vi "Verify Checksum.vi"(6 "error in (no error)":errorcluster, 8 "Input Cmd":string) -> (0 "error out":errorcluster, 2 "Trimmed String":string)   [LabVIEW 2013, in "TDK-Lambda Z.lvlib"]
doc: "This VI will add a checksum to any command string.\nThe format of the \"ChkSum Cmd\" output is:\n \"Command\" & \"Dollar Sign\" & \"Two Hex Digits\" & \"Carriage Return\"\n\nThe command is only formulated, it is not sent to the instrument.\n\nVerify the \"$xx\" checksum which was appended to end of any response string"
uses:
  TDK-Lambda Z.lvlib
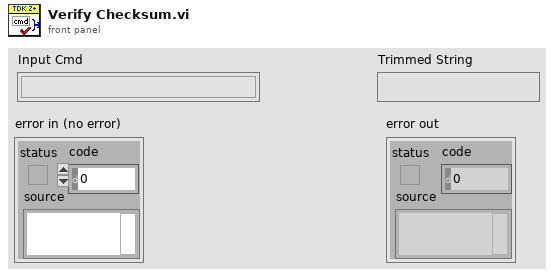
[diagram p1: front panel]
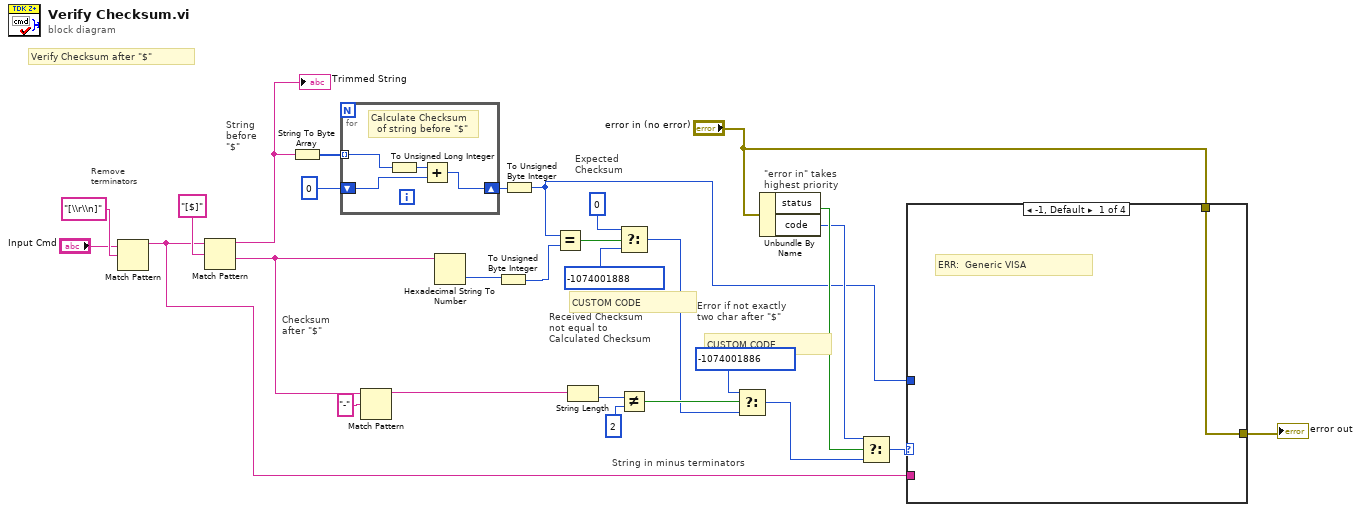
[diagram p0: block diagram]
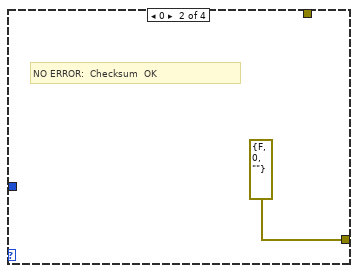
[diagram p2: hidden frame]
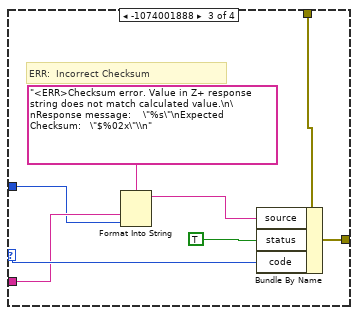
[diagram p3: hidden frame]
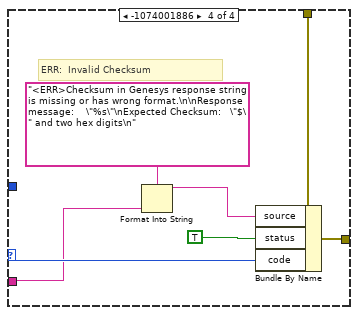
[diagram p4: hidden frame]
diagram:
  # "Expected\nChecksum"
  # "String in minus terminators"
  # "\"error in\" takes\nhighest priority"
  # "String\nbefore\n\"$\""
  # "Checksum\nafter \"$\""
  # "CUSTOM CODE"
  # "Received Checksum\nnot equal to\nCalculated Checksum"
  # "Error if not exactly\ntwo char after \"$\""
  # "CUSTOM CODE"
  # "Remove\nterminators"
  # "Verify Checksum after \"$\""
  n1 = Match Pattern(string="Input Cmd", regular expression="[\\r\\n]") -> (before substring=w9:string)  [unwired: 1 in, 3 out]
  n2 = Match Pattern(string=w9, regular expression="[$]") -> (before substring=w10:string, after substring=w3:string)  [unwired: 1 in, 2 out]
  "Trimmed String" <- w10
  n3 = String To Byte Array(string=w10) -> (unsigned byte array=w27:u8[])
  n4 = for {
    tunnel: w27 -> [w32] mode=indexing
    shift-right: [w30] -> w8
    shift-left: u32 0 -> [w31]
    # "Calculate Checksum\n  of string before \"$\""
    n5 = To Unsigned Long Integer(number=w32) -> (unsigned 32bit integer=w29:u32)
    n6 = Add(x=w29, y=w31) -> (x+y=w30:u32)
  }
  n7 = Match Pattern(string=w3, regular expression="-") -> (before substring=w1:string)  [unwired: 1 in, 3 out]
  n8 = Hexadecimal String To Number(string=w3) -> (number=w20:u32)  [unwired: 2 in, 1 out]
  n9 = To Unsigned Byte Integer(number=w20) -> (unsigned 8bit integer=w19:u8)
  n10 = To Unsigned Byte Integer(number=w8) -> (unsigned 8bit integer=w7:u8)
  n11 = Equal?(x=w7, y=w19) -> (x = y?=w18:bool)
  n12 = String Length(string=w1) -> (length=w24:i32)
  n13 = Select(t=0 ("code"), s=w18, f=-1074001888 ("code")) -> (s? t:f=w16:i32)
  n14 = Not Equal?(x=w24, y=2) -> (x != y?=w22:bool)
  n15 = Select(t=-1074001886 ("code"), s=w22, f=w16) -> (s? t:f=w12:i32)
  n16 = Unbundle By Name("error in (no error)") -> ("status"=w14:bool, "code"=w13:i32)
  n17 = Select(t=w13, s=w14, f=w12) -> (s? t:f=w11:i32)
  n18 = case shown="-1, Default" w11 {
    selector: w11 -> [_ _ w40 w46]
    tunnel: "error in (no error)" -> [w33 _ w41 w48]
    tunnel: [w33 errorcluster {"status"=FALSE, "code"=0, "source"=""} ("error IO") w37 w47] -> w4
    tunnel: w9 -> [_ _ w39 w43]
    tunnel: w7 -> [_ _ w38 _]
    frame -1, Default {
      # "ERR:  Generic VISA"
    }
    frame 0 {
      # "NO ERROR:  Checksum  OK"
    }
    frame -1074001888 {
      # "ERR:  Incorrect Checksum"
      n19 = Format Into String(format string="<ERR>Checksum error. Value in Z+ response string does not match calculated value.\n\nResponse message:    \"%s\"\nExpected Checksum:   \"$%02x\"\\n" ("Source (VI Name)"), w39, w38) -> (resulting string=w36:string)  [unwired: 2 in, 1 out]
      n20 = Bundle By Name(cluster=w41, "source"=w36, "status"=TRUE, "code"=w40) -> (w37:errorcluster)
    }
    frame -1074001886 {
      # "ERR:  Invalid Checksum"
      n21 = Format Into String(format string="<ERR>Checksum in Genesys response string is missing or has wrong format.\n\nResponse message:    \"%s\"\nExpected Checksum:   \"$\" and two hex digits\n" ("Source (VI Name)"), w43) -> (resulting string=w44:string)  [unwired: 2 in, 1 out]
      n22 = Bundle By Name(cluster=w48, "source"=w44, "status"=TRUE, "code"=w46) -> (w47:errorcluster)
    }
  }
  "error out" <- w4
